vi "TimeFormatTry.vi"() -> ()   [LabVIEW 2012]
uses:
  <vilib>/addons/database/Connection.llb/DB Tools Open Connec (Path).vi
  <vilib>/addons/database/NI_Database_API.lvlib
  SQL project lib.lvlib
panel:
  out "SQL format date-time string":string
  out "current time":timestamp
  in  "Numeric 18":dbl
  in  "Numeric 17":dbl
  in  "Numeric 16":dbl
  in  "Numeric 15":dbl
  in  "Numeric 14":dbl
  in  "Numeric 10":dbl
  in  "Numeric 9":dbl
  in  "Numeric 8":dbl
  in  "Numeric 7":dbl
  in  "Numeric 6":dbl
  in  "Numeric 5":dbl
  in  "Numeric 4":dbl
  in  "Numeric 3":dbl
  in  "Numeric 2":dbl
  in  "stop":bool
  out "date/time string":string
  in  "Table Name (The table that you want to save the data into)":string="exodata"
  in  "Numeric":dbl
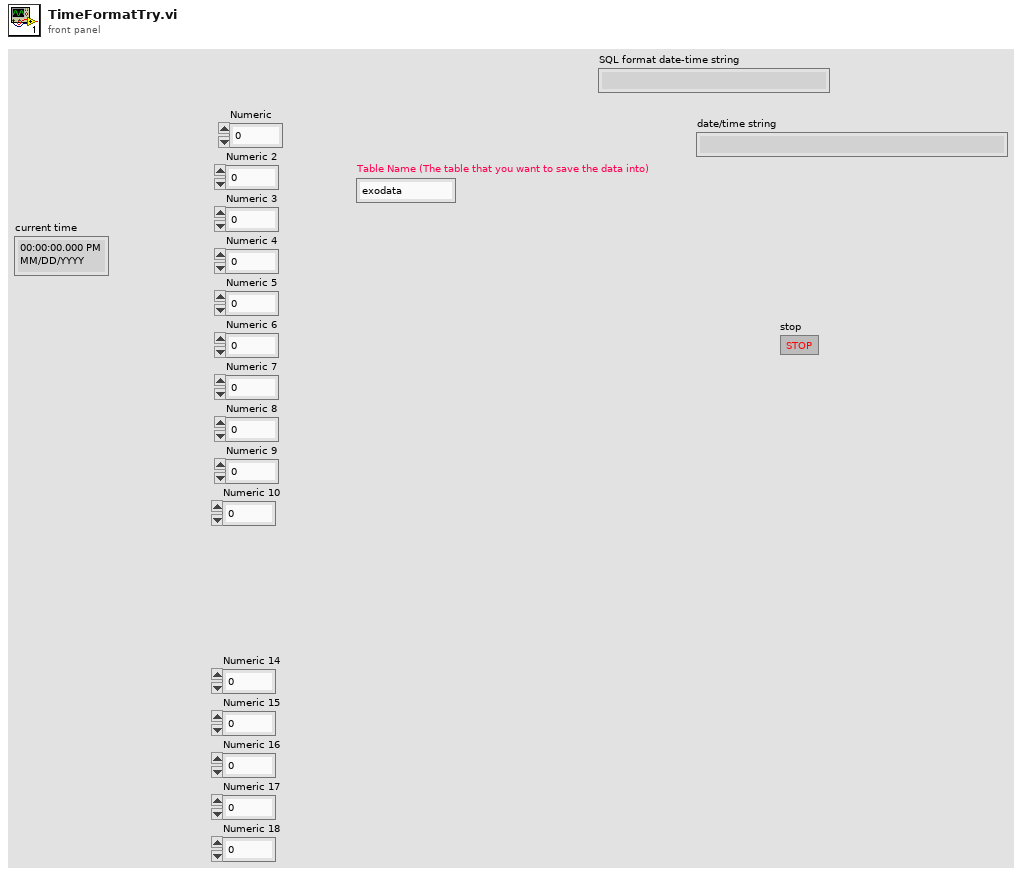
[diagram p1: front panel]
types:
  T1 = cluster{"SQL format date-time string":string, sgl, sgl, sgl, sgl, sgl, sgl, sgl, sgl, sgl, sgl, sgl, sgl, sgl, sgl, sgl, sgl, sgl, sgl}
  T2 = typedef "NI_Database_API.lvlib/Conn ObjectReference.ctl" = refnum<k1>
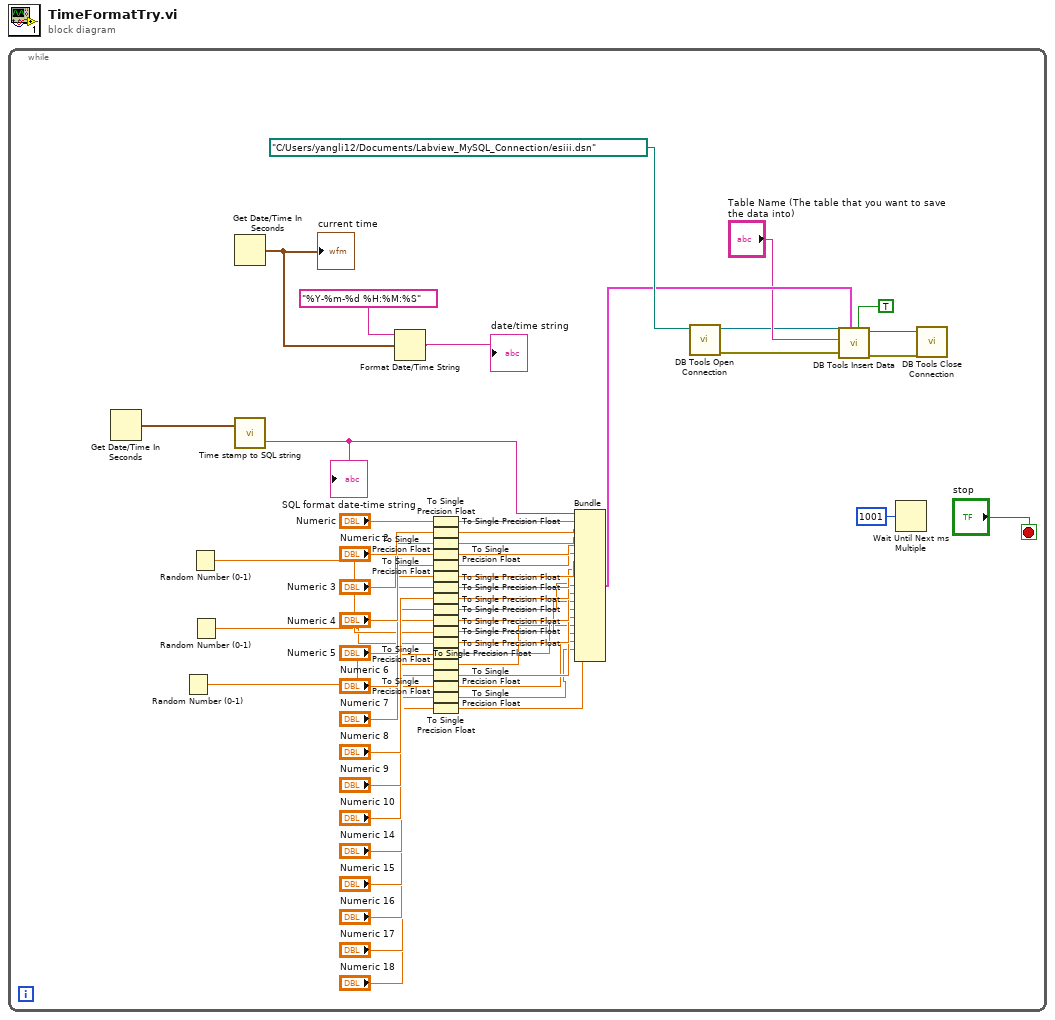
[diagram p0: block diagram]
diagram:
  n1 = while {
    stop <- "stop" stop-if-true
    n2 = Get Date/Time In Seconds() -> (seconds since 1Jan1904=w2:timestamp)
    n3 = Random Number (0-1)() -> (number: 0 to 1=w6:dbl)
    n4 = Random Number (0-1)() -> (number: 0 to 1=w8:dbl)
    n5 = Random Number (0-1)() -> (number: 0 to 1=w7:dbl)
    n6 = Get Date/Time In Seconds() -> (seconds since 1Jan1904=w5:timestamp)
    "current time" <- w5
    n7 = call "Time stamp to SQL string.vi"("time stamp"=w2) -> ("SQL format date-time string"=w1:string)  [unwired: 1 in, 1 out]
    "SQL format date-time string" <- w1
    n8 = Format Date/Time String(time format string (%c)="%Y-%m-%d %H:%M:%S", seconds (now)=w5) -> (date/time string=→"date/time string":string)  [unwired: 1 in]
    n9 = To Single Precision Float(number="Numeric") -> (single precision float=w42:sgl)
    n10 = To Single Precision Float(number="Numeric 2") -> (single precision float=w30:sgl)
    n11 = To Single Precision Float(number="Numeric 3") -> (single precision float=w29:sgl)
    n12 = To Single Precision Float(number="Numeric 4") -> (single precision float=w28:sgl)
    n13 = To Single Precision Float(number="Numeric 5") -> (single precision float=w27:sgl)
    n14 = To Single Precision Float(number="Numeric 6") -> (single precision float=w26:sgl)
    n15 = To Single Precision Float(number="Numeric 7") -> (single precision float=w25:sgl)
    n16 = To Single Precision Float(number="Numeric 8") -> (single precision float=w24:sgl)
    n17 = To Single Precision Float(number="Numeric 9") -> (single precision float=w23:sgl)
    n18 = To Single Precision Float(number="Numeric 10") -> (single precision float=w22:sgl)
    n19 = To Single Precision Float(number=w8) -> (single precision float=w21:sgl)
    n20 = To Single Precision Float(number=w7) -> (single precision float=w20:sgl)
    n21 = To Single Precision Float(number=w6) -> (single precision float=w19:sgl)
    n22 = To Single Precision Float(number="Numeric 14") -> (single precision float=w13:sgl)
    n23 = To Single Precision Float(number="Numeric 15") -> (single precision float=w12:sgl)
    n24 = To Single Precision Float(number="Numeric 16") -> (single precision float=w11:sgl)
    n25 = To Single Precision Float(number="Numeric 17") -> (single precision float=w10:sgl)
    n26 = To Single Precision Float(number="Numeric 18") -> (single precision float=w9:sgl)
    n27 = Bundle("SQL format date-time string"=w1, w42, w30, w29, w28, w27, w26, w25, w24, w23, w22, w21, w20, w19, w13, w12, w11, w10, w9) -> (w50:T1)  [unwired: 1 in]
    n28 = call-poly <vilib>:"DB Tools Open Connection.vi"("connection information"=path "C:/Users/yangli12/Documents/Labview_MySQL_Connection/esiii.dsn") -> ("error out"=w47:errorcluster, "connection reference"=w48:T2)  [unwired: 7 in]
    n29 = call <vilib>:"DB Tools Insert Data.vi"("create table? (F)"=TRUE, "data"=w50, "error in (no error)"=w47, "table"="Table Name (The table that you want to save the data into)", "connection reference"=w48) -> ("error out"=w45:errorcluster, "connection reference out"=w46:T2)  [unwired: 5 in]
    n30 = Wait Until Next ms Multiple(millisecond multiple=u32 1001) -> ()  [unwired: 1 out]
    n31 = call <vilib>:"DB Tools Close Connection.vi"("error in (no error)"=w45, "connection reference"=w46) -> ()  [unwired: 5 in, 1 out]
  }
